vi "Compile Asynchronous Execution Units.vi"(0 "Device Ref in":T2=18446744073709551615 format="%.0x", 1 "Asynchronous Execution Units":T3[](array[typedef]) {"ReadWrite Channels" format="%.0x"; "Outgoing Channels" format="%.0x"; "Incoming Channels" format="%.0x"}, 3 "error in":errorcluster) -> (7 "Device Ref out":T2=18446744073709551615 format="%.0x", 8 "Compiled Asynchronous Execution Units":T1[](array[typedef]), 10 "error out":errorcluster)   [LabVIEW 2020, in "Communication Bus Template System Explorer.lvlib"]
uses:
  Communication Bus Template System Explorer.lvlib
  Includes/Communication Bus Engine.lvlibp/Engine/Interfaces/Controls/Execution Unit Information.ctl
  Includes/Communication Bus Engine.lvlibp/Engine/Interfaces/Execution Unit/Execution Unit.lvclass
  Includes/Communication Bus Engine.lvlibp/1abvi3w/vi.lib/NI VeriStand/Custom Device API/Custom Device Item Ref.ctl
  <vilib>/NI VeriStand/Custom Device API/Custom Device Item Ref.ctl
  Shared/Asynchronous Execution Unit Compiled Information.ctl
  <vilib>/NI VeriStand/Custom Device API/Custom Device API.lvlib
  <vilib>/NI/NIVS Inline Async API/_Data Access System Explorer/Data Access System Explorer.lvlib
  Shared/Communication Bus Template Shared.lvlib
  Includes/Communication Bus Engine.lvlibp/1abvi3w/vi.lib/NI VeriStand/Custom Device API/Custom Device API.lvlib
  Includes/Communication Bus Engine.lvlibp/Engine/Interfaces/Interfaces.lvlib
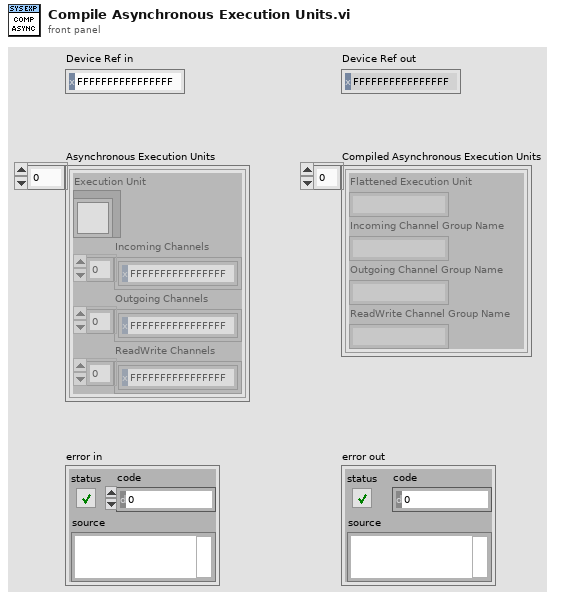
[diagram p1: front panel]
types:
  T1 = typedef "Communication Bus Template Shared.lvlib/Asynchronous Execution Unit Compiled Information.ctl" = cluster{"Flattened Execution Unit":string, "Incoming Channel Group Name":string, "Outgoing Channel Group Name":string, "ReadWrite Channel Group Name":string}
  T2 = typedef "Custom Device API.lvlib/Custom Device Item Ref.ctl" = u64
  T3 = typedef "Communication Bus Engine.lvlibp/Interfaces.lvlib/Execution Unit Information.ctl" = cluster{"Execution Unit":refnum<class "Execution Unit.lvclass">, "Incoming Channels":T4[], "Outgoing Channels":T4[], "ReadWrite Channels":T4[]}
  T4 = typedef "Communication Bus Engine.lvlibp/Custom Device API.lvlib/Custom Device Item Ref.ctl" = u64
  T5 = enum16{"Output/Write", "Input/Read", "Input/ReadWrite"}
  T6 = cluster{"Name":string, "Type":enum16{"Output/Write", "Input/Read", "Input/ReadWrite"}, "VS Refs":T2[]}
  T7 = cluster{"Name":string, "Type":enum16{"Output/Write", "Input/Read", "Input/ReadWrite"}, "VS Refs":T2[]}[]
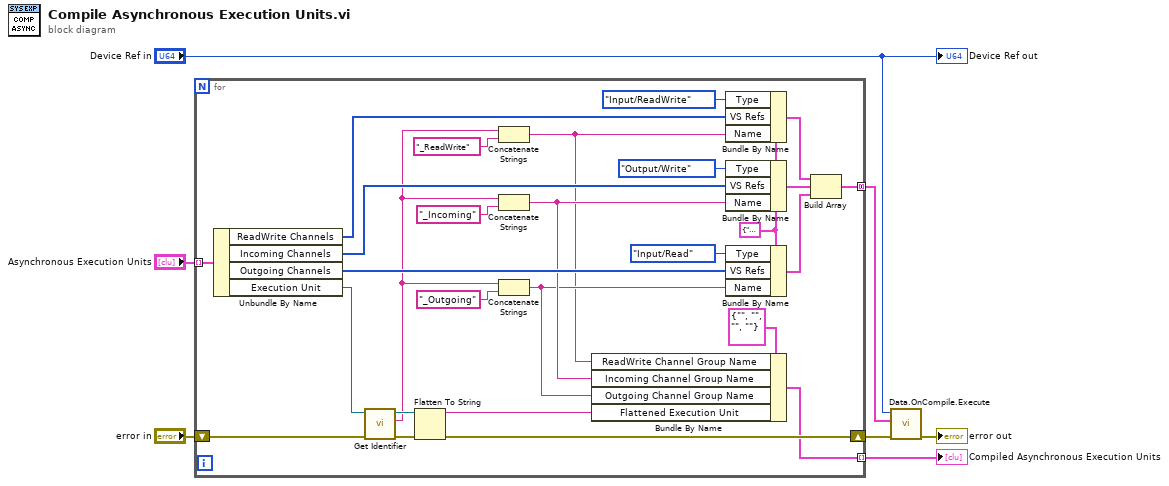
[diagram p0: block diagram]
diagram:
  n1 = for {
    tunnel: "Asynchronous Execution Units" -> [w33] mode=indexing
    tunnel: [w26] -> w6 mode=concatenating
    shift-right: [w25] -> w2
    shift-left: "error in" -> [w24]
    tunnel: [w19] -> w1 mode=indexing
    w15 = T6 {"Name"="", "Type"=enum."Output/Write", "VS Refs"=[]} ("Group")
    n2 = Unbundle By Name(w33) -> ("ReadWrite Channels"=w13:T4[], "Incoming Channels"=w34:T4[], "Outgoing Channels"=w28:T4[], "Execution Unit"=w22:refnum<class "Execution Unit.lvclass">)
    n3 = call-dynamic "Get Identifier.vi"("error in (no error)"=w24, "Execution Unit in"=w22) -> ("error out"=w23:errorcluster, "Identifier"=w11:string, "Execution Unit out"=w21:refnum<class "Execution Unit.lvclass">)  [unwired: 7 in]
    n4 = Flatten To String(anything=w21, error in (no error)=w23) -> (data string=w10:string, error out=w25:errorcluster)  [unwired: 2 in, 1 out]
    n5 = Concatenate Strings(w11, "_ReadWrite" ("string")) -> (w9:string)
    n6 = Concatenate Strings(w11, "_Incoming" ("string")) -> (w18:string)
    n7 = Concatenate Strings(w11, "_Outgoing" ("string")) -> (w17:string)
    n8 = Bundle By Name(cluster=T1 {"Flattened Execution Unit"="", "Incoming Channel Group Name"="", "Outgoing Channel Group Name"="", "ReadWrite Channel Group Name"=""} ("Asynchronous Execution Unit Compiled Information"), "ReadWrite Channel Group Name"=w9, "Incoming Channel Group Name"=w18, "Outgoing Channel Group Name"=w17, "Flattened Execution Unit"=w10) -> (w19:T1)
    n9 = Bundle By Name(cluster=w15, "Type"=T5."Input/ReadWrite", "VS Refs"=w13, "Name"=w9) -> (w8:T6)
    n10 = Bundle By Name(cluster=w15, "Type"=T5."Output/Write", "VS Refs"=w34, "Name"=w18) -> (w16:T6)
    n11 = Bundle By Name(cluster=w15, "Type"=T5."Input/Read", "VS Refs"=w28, "Name"=w17) -> (w27:T6)
    n12 = Build Array(w8, w16, w27) -> (w26:T7)
  }
  "Compiled Asynchronous Execution Units" <- w1
  n13 = call <vilib>:"Data.OnCompile.Execute.vi"("error in"=w2, "VS Ref Groups"=w6, "Custom Device Ref"="Device Ref in") -> ("error out"=→"error out":errorcluster)  [unwired: 7 in, 1 out]
  "Device Ref out" <- "Device Ref in"
